vi "난수발생.vi"() -> ()   [LabVIEW 2014]
panel:
  in  "path to BMP file":path=path "C:/Users/lvedu/Desktop/b.bmp" caption="BMP 파일 경로"
  in  "경로":path
  in  "가운데로":bool
  in  "메뉴바/도구바":bool
  in  "정지":bool
  in  "난수 발생":bool
  out "웨이브폼 차트":dbl(graph)
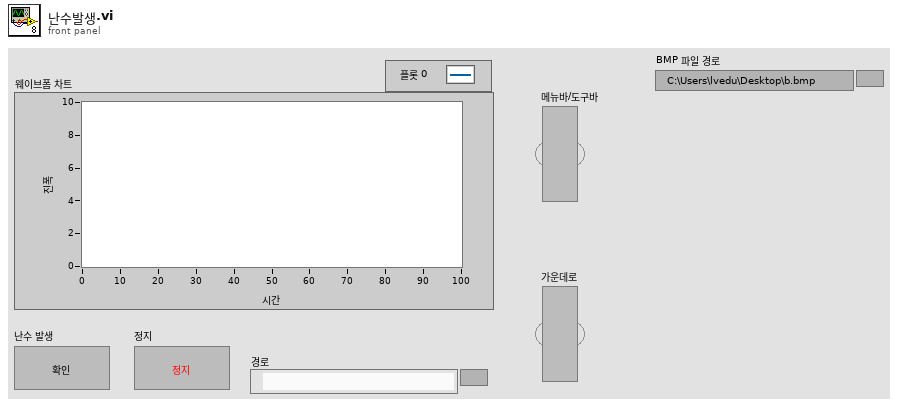
[diagram p1: front panel]
types:
  T1 = cluster{"left":i16, "top":i16, "right":i16, "bottom":i16}
  T2 = enum16{"Always On", "Always Off", "Off While Running"}
  T3 = typedef "imagedata.ctl" = cluster{"image type":i32, "image depth":i32, "image":u8[], "mask":u8[], "colors":u32[], "Rectangle":cluster{"left":i16, "top":i16, "right":i16, "bottom":i16}}
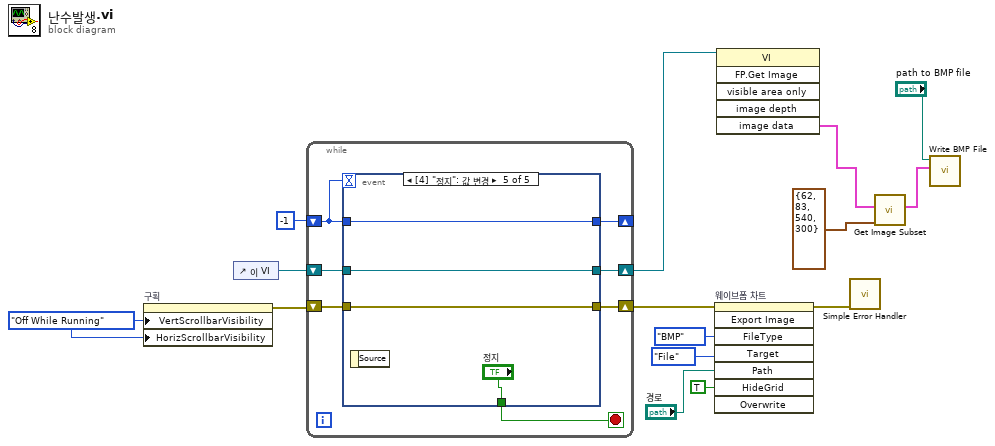
[diagram p0: block diagram]
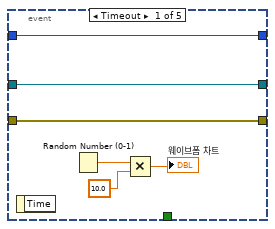
[diagram p2: hidden frame]
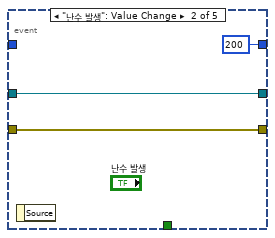
[diagram p3: hidden frame]
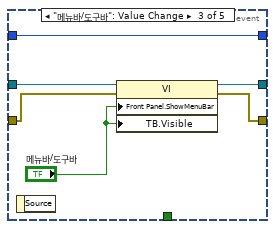
[diagram p4: hidden frame]
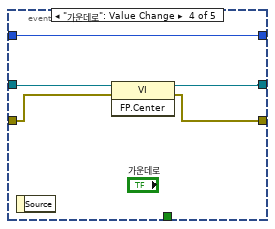
[diagram p5: hidden frame]
diagram:
  w13 = T2."Off While Running" ("수직 스크롤 막대 보이기")
  n1 = property on="구획" class="Pane"("VertScrollbarVisibility"=w13, "HorizScrollbarVisibility"=w13) -> (error out=w12:errorcluster)  [unwired: 2 in, 1 out]
  n2 = control-ref of="이 VI"() -> (w14:refnum<vi>)
  n3 = while {
    shift-right: [w21] -> _
    shift-left: -1 -> [w22]
    shift-right: [w17] -> w1
    shift-left: w14 -> [w19]
    shift-right: [w16] -> w11
    shift-left: w12 -> [w18]
    stop <- w20 stop-if-true
    n4 = event shown="[4] \"정지\": 값 변경" {
      selector: _ -> [_ _ _ _ _]
      dyn-events: _ -> [_ _ _ _ _]
      timeout: w22 -> [_ _ _ _ _]
      tunnel: [w28 200 w37 w42 w45] -> w21
      tunnel: w22 -> [w28 _ w37 w42 w45]
      tunnel: [_ _ _ _ "정지"] -> w20
      tunnel: w19 -> [w24 w31 w35 w41 w44]
      tunnel: w18 -> [w23 w30 w34 w39 w43]
      tunnel: [w24 w31 w36 w40 w44] -> w17
      tunnel: [w23 w30 w33 w38 w43] -> w16
      event Timeout {
        n5 = event-data() -> ()  [unwired: 1 in, 1 out]
        n6 = Random Number (0-1)() -> (number: 0 to 1=w26:dbl)
        n7 = Multiply(x=w26, y=10.0) -> (x*y=→"웨이브폼 차트":dbl)
      }
      event "난수 발생": Value Change {
        n8 = event-data() -> ()  [unwired: 1 in, 1 out]
      }
      event "메뉴바/도구바": Value Change {
        n9 = event-data() -> ()  [unwired: 1 in, 1 out]
        n10 = property class="VI"(reference=w35, error in=w34, "Front Panel.ShowMenuBar"="메뉴바/도구바", "TB.Visible"="메뉴바/도구바") -> (reference out=w36:refnum<vi>, error out=w33:errorcluster)
      }
      event "가운데로": Value Change {
        n11 = event-data() -> ()  [unwired: 1 in, 1 out]
        n12 = invoke class="VI" method="FP.Center"(reference=w41, error in=w39) -> (reference out=w40:refnum<vi>, error out=w38:errorcluster)  [unwired: 1 in, 1 out]
      }
      event "정지": Value Change {
        n13 = event-data() -> ()  [unwired: 1 in, 1 out]
      }
    }
  }
  n14 = invoke on="웨이브폼 차트" class="WFChart (엄격한)" method="Export Image"(error in=w11, "FileType"=enum32{"BMP", "EPS", "EMF", "PICT"}."BMP" ("파일 타입"), "Target"=enum32{"File", "Clipboard"}."File" ("타겟"), "Path"="경로", "HideGrid"=TRUE ("눈금 숨기기")) -> (error out=w6:errorcluster)  [unwired: 3 in, 7 out]
  n15 = invoke class="VI" method="FP.Get Image"(reference=w1) -> ("image data"=w4:T3)  [unwired: 5 in, 5 out]
  n16 = call <vilib>:"Simple Error Handler.vi"("error in (no error)"=w6) -> ()  [unwired: 4 in, 5 out]
  n17 = call <vilib>:"Get Image Subset.vi"("subset rect"=T1 {"left"=62, "top"=83, "right"=540, "bottom"=300}, "image data"=w4) -> ("image subset"=w3:T3)  [unwired: 4 in, 1 out]
  n18 = call <vilib>:"Write BMP File.vi"("image data"=w3, "path to BMP file"="path to BMP file") -> ()  [unwired: 8 in, 2 out]
